vi "test Acyclic Loopback.vi"(8 "error in":errorcluster, 11 "TestCase in":refnum<class "Single Board Loopback.lvclass">) -> (0 "error out":errorcluster, 3 "TestCase out":refnum<class "Single Board Loopback.lvclass">)   [LabVIEW 2020, in "Single Board Loopback.lvclass"]
uses:
  Single Board Loopback.lvclass
  C:/dev/git/niveristand-custom-device-testing-tools/VeriStandTestCase/VeriStandTestCase.lvclass
  <vilib>/numeric/Random Number (Range) U64.vi
  <vilib>/numeric/sub_Random U32.vi
  <vilib>/NI VeriStand/Execution/Workspace/NI VeriStand - Set Multiple Channel Values.vi
  <vilib>/addons/_JKI Toolkits/VI Tester/TestCase.llb/TestCase.lvclass
  <vilib>/NI VeriStand/Execution/Workspace/NI_VS Workspace ExecutionAPI.lvlib
  niveristand-custom-device-testing-tools/VeriStandTestUtilities/VeriStandTestUtilities.lvlib
  C:/Program Files (x86)/National Instruments/LabVIEW 2020/vi.lib/addons/_JKI Toolkits/VI Tester/TestCase.llb/TestCase.lvclass
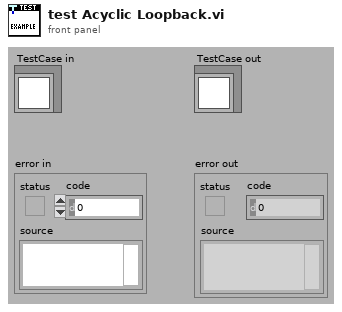
[diagram p1: front panel]
types:
  T1 = typedef "NI_VS Workspace ExecutionAPI.lvlib/WorkspaceAPI.ctl" = refnum<k24>
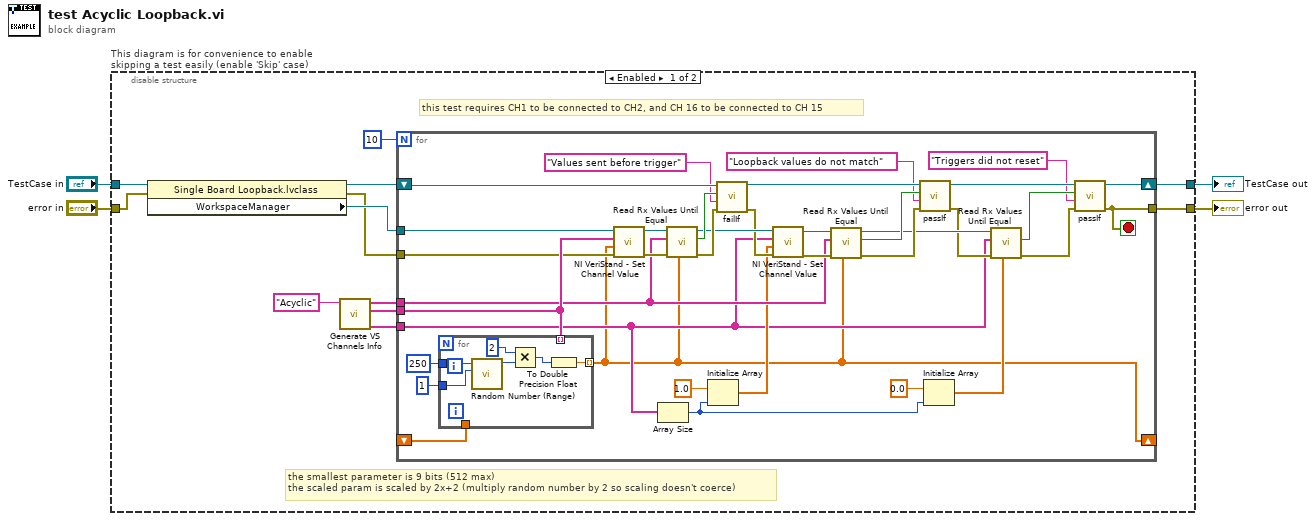
[diagram p0: block diagram]
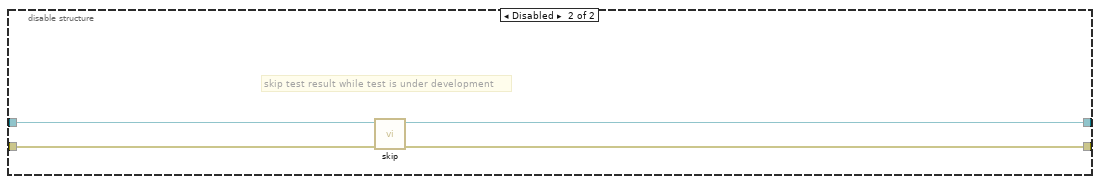
[diagram p2: hidden frame]
diagram:
  n1 = disable-structure "This diagram is for convenience to enable skipping a test easily (enable 'Skip' case)" shown="Enabled" {
    disable-tunnel: "TestCase in" -> [w11 w62]
    disable-tunnel: [w9 w60] -> w1
    disable-tunnel: [w8 w61] -> w3
    disable-tunnel: "error in" -> [w10 w59]
    frame Enabled {
      # "this test requires CH1 to be connected to CH2, and CH 16 to be connected to CH 15"
      # "the smallest parameter is 9 bits (512 max)\nthe scaled param is scaled by 2x+2 (multiply random number by 2 so scaling doesn't coerce)"
      n2 = property class="Single Board Loopback.lvclass"(reference=w11, error in=w10) -> (reference out=w13:refnum<class "Single Board Loopback.lvclass">, error out=w14:errorcluster, "WorkspaceManager"=w15:T1)
      n3 = call "Generate VS Channels Info.vi"("Transfer Type"="Acyclic") -> ("Tx Trigger Channels Array"=w6:string[], "Tx Channels Array"=w7:string[], "Rx Channels Array"=w16:string[])  [unwired: 6 in, 2 out]
      n4 = for {
        N: 10 -> [_]
        tunnel: w16 -> [w38]
        tunnel: w15 -> [w50]
        tunnel: w14 -> [w43]
        tunnel: w7 -> [w49]
        shift-right: [w32] -> w9
        shift-left: w13 -> [w45]
        tunnel: [w34] -> w8
        tunnel: w6 -> [w22]
        shift-right: [w18] -> _
        shift-left: _ -> [w17]
        stop <- w34 stop-if-true
        n5 = for {
          tunnel: [w57] -> w18 mode=indexing
          tunnel: u64 250 ("upper bound (100)") -> [w56]
          tunnel: u64 1 ("upper bound (100)") -> [w55]
          tunnel: w49 -> [_] mode=indexing
          tunnel: w17 -> [_]
          n6 = call-poly <vilib>:"Random Number (Range).vi"("lower bound (0)"=w55, "upper bound (100)"=w56) -> ("number"=w58:u64)  [unwired: 9 in]
          n7 = Multiply(x=u64 2, y=w58) -> (x*y=w54:u64)
          n8 = To Double Precision Float(number=w54) -> (double precision float=w57:dbl)
        }
        n9 = call-poly <vilib>:"NI VeriStand - Set Channel Value.vi"("error in (no error)"=w43, "Values"=w18, "Channels"=w49, "WorkspaceManager in"=w50) -> ("error out"=w46:errorcluster, "WorkspaceManager out"=w48:T1)  [unwired: 6 in]
        n10 = Array Size(array=w22) -> (size(s)=w19:i32)
        n11 = call "Read Rx Values Until Equal.vi"("expected values"=w18, "error in"=w46, "Rx aliases"=w38, "workspace manager in"=w48) -> ("error out"=w47:errorcluster, "values equal expected"=w44:bool, "workspace manager out"=w42:T1)  [unwired: 5 in]
        n12 = Initialize Array(1.0, w19) -> (w23:dbl[])
        n13 = call-dynamic "failIf.vi"("error in (no error)"=w47, "message (\"\")"="Values sent before trigger" ("message (\"\")"), "fail"=w44, "TestCase in"=w45) -> ("error out"=w41:errorcluster, "TestCase out"=w35:refnum<class "Single Board Loopback.lvclass">)  [unwired: 6 in]
        n14 = call-poly <vilib>:"NI VeriStand - Set Channel Value.vi"("error in (no error)"=w41, "Values"=w23, "Channels"=w22, "WorkspaceManager in"=w42) -> ("error out"=w39:errorcluster, "WorkspaceManager out"=w40:T1)  [unwired: 6 in]
        n15 = call "Read Rx Values Until Equal.vi"("expected values"=w18, "error in"=w39, "Rx aliases"=w38, "workspace manager in"=w40) -> ("error out"=w36:errorcluster, "values equal expected"=w37:bool, "workspace manager out"=w30:T1)  [unwired: 5 in]
        n16 = call-dynamic "passIf.vi"("error in (no error)"=w36, "message (\"\")"="Loopback values do not match" ("message (\"\")"), "pass"=w37, "TestCase in"=w35) -> ("error out"=w29:errorcluster, "TestCase out"=w33:refnum<class "Single Board Loopback.lvclass">)  [unwired: 6 in]
        n17 = Initialize Array(0.0, w19) -> (w20:dbl[])
        n18 = call "Read Rx Values Until Equal.vi"("expected values"=w20, "error in"=w29, "Rx aliases"=w22, "workspace manager in"=w30) -> ("error out"=w28:errorcluster, "values equal expected"=w31:bool)  [unwired: 5 in, 1 out]
        n19 = call-dynamic "passIf.vi"("error in (no error)"=w28, "message (\"\")"="Triggers did not reset" ("message (\"\")"), "pass"=w31, "TestCase in"=w33) -> ("error out"=w34:errorcluster, "TestCase out"=w32:refnum<class "Single Board Loopback.lvclass">)  [unwired: 6 in]
      }
    }
    frame Disabled {
      # "skip test result while test is under development"
      n20 = call <vilib>:"skip.vi"("error in (no error)"=w59, "TestCase in"=w62) -> ("error out"=w61:errorcluster, "TestCase out"=w60:refnum<class "Single Board Loopback.lvclass">)  [unwired: 8 in]
    }
  }
  "error out" <- w3
  "TestCase out" <- w1
